vi "Anritsu VNA Set Trace.vi"(7 "Anritsu VNA":T1, 8 "error in (no error)":errorcluster, 9 "Trace":i8=1 min=1 max=99 step=1, 10 "Channel":i8=1 min=1 max=99 step=1, 11 "VISA Resource Name":refnum<visa-resource-name>) -> (0 "error out":errorcluster, 3 "dup VISA Resource Name":refnum<visa-resource-name>)   [LabVIEW 2011]
uses:
  TypeDefs/Anritsu VNA Instrument Info.ctl
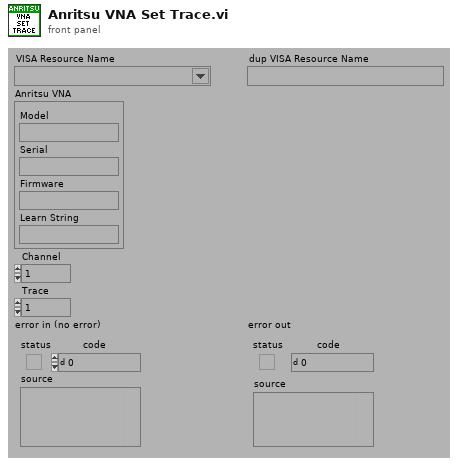
[diagram p1: front panel]
types:
  T1 = typedef "Anritsu VNA Instrument Info.ctl" = cluster{"Model":string, "Serial":string, "Firmware":string, "Learn String":string}
  T2 = typedef "Anritsu VNA Model.ctl" = enum16{"Not Supported", "37XXXX", "MS20XXX", "MS462XX", "MS464XX"}
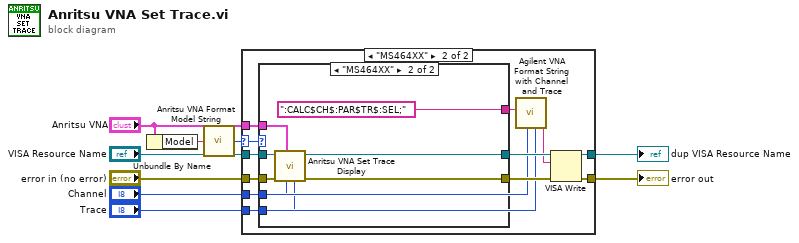
[diagram p0: block diagram]
diagram:
  n1 = Unbundle By Name("Anritsu VNA") -> ("Model"=w3:string)
  n2 = call "Anritsu VNA Format Model String.vi"("Model"=w3) -> ("Model"=w1:T2)
  n3 = case shown="\"MS464XX\"" w1 {
    selector: w1 -> [_ w12]
    tunnel: [w11 w23] -> w9
    tunnel: [w10 w22] -> w8
    tunnel: "VISA Resource Name" -> [w11 w21]
    tunnel: "error in (no error)" -> [w10 w20]
    tunnel: "Trace" -> [_ w15]
    tunnel: "Channel" -> [_ w14]
    tunnel: "Anritsu VNA" -> [_ w13]
    frame "Not Supported".."MS462XX" {
    }
    frame "MS464XX" {
      n4 = case shown="\"MS464XX\"" w12 {
        tunnel: [_ ":CALC$CH$:PAR$TR$:SEL;"] -> w16
        tunnel: w21 -> [w25 w28]
        tunnel: w20 -> [w24 w30]
        tunnel: [w25 w26] -> w19
        tunnel: [w24 w27] -> w18
        tunnel: w13 -> [_ w32]
        tunnel: w14 -> [_ w29]
        tunnel: w15 -> [_ w31]
        frame "Not Supported".."MS462XX" {
        }
        frame "MS464XX" {
          n5 = call "Anritsu VNA Set Trace Display.vi"("Trace"=w31, "Channel"=w29, "Anritsu VNA"=w32, "error in (no error)"=w30, "VISA Resource Name"=w28) -> ("error out"=w27:errorcluster, "dup VISA Resource Name"=w26:refnum<visa-resource-name>)  [unwired: 5 out]
        }
      }
      n6 = call "Agilent VNA Format String with Channel and Trace.vi"("Trace"=w15, "Channel"=w14, "String"=w16) -> ("String Out"=w17:string)  [unwired: 6 out]
      n7 = VISA Write(VISA resource name=w19, write buffer=w17, error in (no error)=w18) -> (VISA resource name out=w23:refnum<visa-resource-name>, error out=w22:errorcluster)  [unwired: 1 out]
    }
  }
  "dup VISA Resource Name" <- w9
  "error out" <- w8
